vi "PositionControlTest.vi"() -> ()   [LabVIEW 2019]
uses:
  <vilib>/myRIO/Common/Instrument Driver Framework/myRIO v1.0/Encoder/typedefs/Encoder Count Direction Enum.ctl
  <vilib>/myRIO/Common/Instrument Driver Framework/myRIO v1.0/Encoder/typedefs/Encoder Signal Mode.ctl
  <vilib>/myRIO/Common/Instrument Driver Framework/myRIO v1.0/Encoder/typedefs/Encoder Channels Enum.ctl
  <vilib>/myRIO/Common/Instrument Driver Framework/Utilities/typedefs/Generic FPGA Reference.ctl
  <vilib>/myRIO/Common/Instrument Driver Framework/Utilities/typedefs/myRIO v1.0 Reference.ctl
  <vilib>/myRIO/Common/Instrument Driver Framework/Utilities/typedefs/Hardware Version Enum.ctl
  <vilib>/myRIO/Common/Instrument Driver Framework/Utilities/typedefs/myRIO Generic Hardware Reference.ctl
  <vilib>/myRIO/Instrument Drivers/Onboard IO/Encoder/typedefs/Encoder Reference.ctl
  <vilib>/myRIO/Instrument Drivers/Onboard IO/Encoder/Encoder.lvlib
  <vilib>/myRIO/Instrument Drivers/Onboard IO/Encoder/vis/Read.vi
  <vilib>/myRIO/Common/Instrument Driver Framework/myRIO v1.0/Encoder/typedefs/Encoder Configuration v1.0.ctl
  <vilib>/userdefined/High Color/nirio_resource_hc.ctl
  <vilib>/myRIO/Common/Instrument Driver Framework/myRIO v1.0/Encoder/vis/myRIO v1.1 Open Encoder.vi
  <vilib>/myRIO/Common/Instrument Driver Framework/myRIO v1.0/Encoder/vis/myRIO v1.0 Configure Encoder.vi
  <vilib>/myRIO/Instrument Drivers/Onboard IO/Encoder/vis/myRIO Encoder Open.xnode
  <vilib>/myRIO/Common/Instrument Driver Framework/Utilities/vis/Is FPGA Ref Available.vi
  <vilib>/myRIO/Express VI/Onboard IO/Encoder/Encoder Express VI.xnode
  <vilib>/Utility/file.llb/Write Delimited Spreadsheet (DBL).vi
  <vilib>/myRIO/Instrument Drivers/Utilities/Utilities.lvlib
panel:
  out "ref pos":dbl
  out "error out 2":errorcluster
  in  "Stop 2":bool
  out "Counter Direction":enum16{"Counting Up", "Counting Down"}(ring)
  out "Overflow?":bool
  in  "Reset Counter":bool
  out "actual pos":dbl
  out "Graph 2":cluster{dbl, dbl}(graph)
  in  "Frequency [Hz]":dbl=1000.0
  out "Duty Cycle":dbl=0.5
  in  "pos ref":dbl(slide) scale=-3.0..3.0
  in  "K":dbl format="%#_13g"
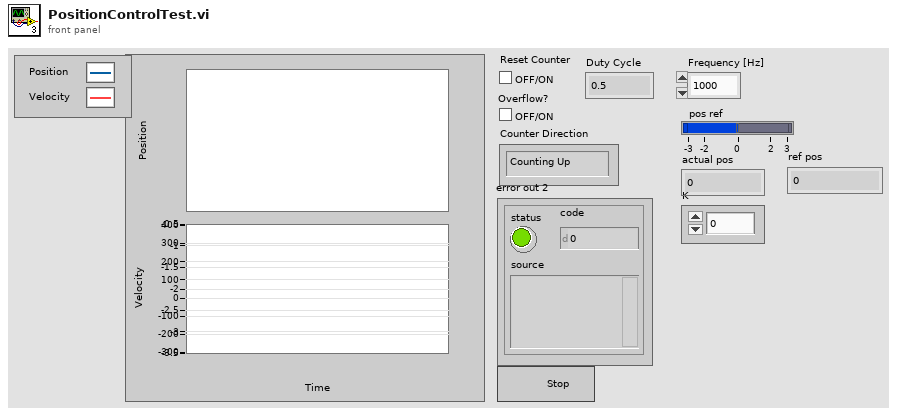
[diagram p1: front panel]
types:
  T1 = typedef "Encoder.lvlib/Encoder Reference.ctl" = cluster{"myRIO Reference":T2, "Encoder Channels Enum":T6}
  T2 = typedef "myRIO Generic Hardware Reference.ctl" = cluster{"myRIO Model":T3, "myRIO Hardware Reference":T4}
  T3 = typedef "Hardware Version Enum.ctl" = enum16{"Unknown", "myRIO-1900", "myRIO-1950", "roboRIO", "NI ELVIS RIO CM", "ELVIS III"}
  T4 = typedef "myRIO v1.0 Reference.ctl" = cluster{"Generic FPGA Reference":T5, "Allow multiple opens":bool}
  T5 = typedef "Generic FPGA Reference.ctl" = refnum<k20>
  T6 = typedef "Encoder Channels Enum.ctl" = enum16{"Not Connected", "C/ENC0", "C/ENC1", "A/ENC", "A/ENC0", "A/ENC1", "A/ENC2", "A/ENC3", "A/ENC4", "A/ENC5", "A/ENC6", "A/ENC7", "A/ENC8", "A/ENC9", "B/ENC", "B/ENC0", "B/ENC1", "B/ENC2", "B/ENC3", "B/ENC4", "B/ENC5", "B/ENC6", "B/ENC7", "B/ENC8", "B/ENC9", "DIO/ENC0", "DIO/ENC1", "DIO/ENC2", "DIO/ENC3", "DIO/ENC4"}
  T7 = typedef "Encoder Signal Mode.ctl" = enum16{"Quadrature phase signal", "Step and direction signal"}
  T8 = typedef "nirio_resource_hc.ctl" = tag
  T9 = typedef "Encoder Count Direction Enum.ctl" = enum16{"Counting Up", "Counting Down"}
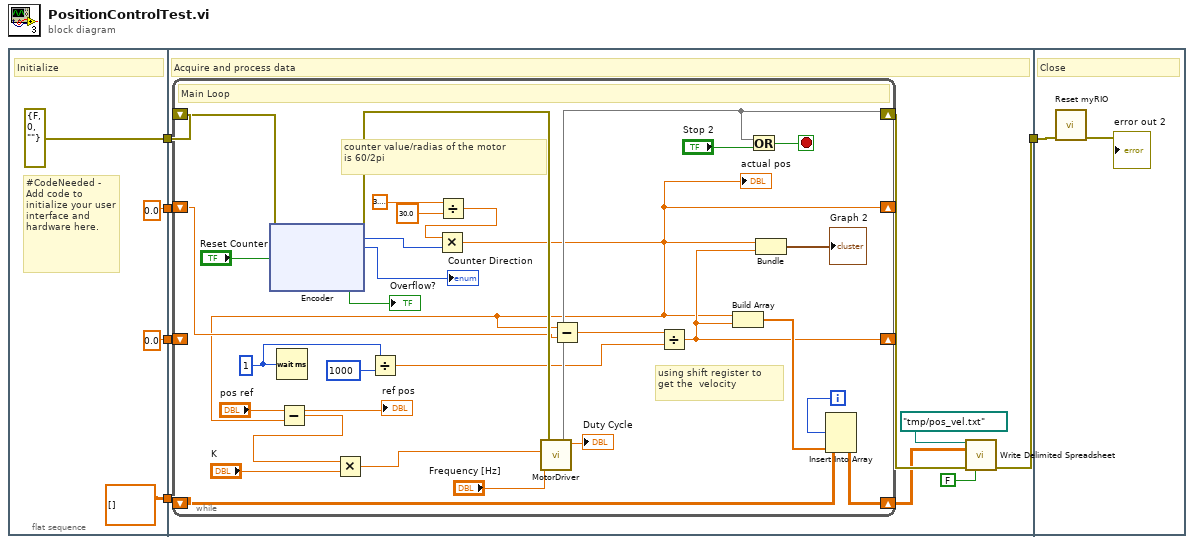
[diagram p0: block diagram]
diagram:
  n1 = flat-sequence {
    tunnel: [errorcluster {"status"=FALSE, "code"=0, "source"=""} ("error in (no error)")] -> w5
    tunnel: [0.0] -> w4
    tunnel: [dbl[][] [] ("array")] -> w3
    tunnel: [0.0] -> w2
    tunnel: w5 -> [w18]
    tunnel: [w13] -> w1
    tunnel: w4 -> [w17]
    tunnel: w3 -> [w16]
    tunnel: w2 -> [w10]
    tunnel: w1 -> [w96]
    frame #0 {
      # "#CodeNeeded - Add code to initialize your user interface and hardware here."
      # "Initialize"
    }
    frame #1 {
      # "Acquire and process data"
      n2 = while {
        shift-right: [w29] -> w14
        shift-left: w18 -> [w26]
        shift-right: [w22] -> _
        shift-left: w17 -> [w24]
        shift-right: [w34] -> w11
        shift-left: w16 -> [w19]
        shift-right: [w28] -> _
        shift-left: w10 -> [_]
        i -> [w35]
        stop <- w47 stop-if-true
        w41 = u32 1 ("milliseconds to wait")
        # "using shift register to\nget the  velocity"
        # "counter value/radias of the motor \nis 60/2pi"
        # "Main Loop"
        n3 = xnode "Encoder"("error in (no error)"=w26, "Reset Counter"="Reset Counter") -> ("error out"=w30:errorcluster, "Counter Value"=w38:i32, "Counter Direction"=→"Counter Direction":T9, "Overflow?"=→"Overflow?":bool)
        n4 = Wait (ms)(milliseconds to wait=w41) -> ()  [unwired: 1 out]
        n5 = Divide(x=w41, y=u32 1000) -> (x/y=w27:dbl)
        n6 = Divide(x=3.141592653589793, y=30.0) -> (x/y=w37:dbl)
        n7 = Multiply(x=w37, y=w38) -> (x*y=w22:dbl)
        "actual pos" <- w22
        n8 = Subtract(x="pos ref", y=w22) -> (x-y=w21:dbl)
        n9 = Multiply(x=w21, y="K") -> (x*y=w20:dbl)
        n10 = call "MotorDriver.vi"("error in (no error)"=w30, "Duty Cycle in"=w20, "Frequency [Hz]"="Frequency [Hz]") -> (0:w29, "Duty Cycle out"=→"Duty Cycle":dbl)  [unwired: 7 in]
        n11 = Subtract(x=w22, y=w24) -> (x-y=w39:dbl)
        n12 = Divide(x=w39, y=w27) -> (x/y=w28:dbl)
        n13 = Build Array(w22, w28) -> (w33:dbl[])
        n14 = Or(x=w29, y="Stop 2") -> (x .or. y?=w47:bool)
        n15 = Bundle(w22, w28) -> (→"Graph 2":cluster{dbl, dbl})  [unwired: 1 in]
        n16 = Insert Into Array(array=w19, index (row)=w35, new element=w33) -> (w34:dbl[][])  [unwired: 1 in]
        "ref pos" <- "pos ref"
      }
      n17 = call-poly <vilib>:"Write Delimited Spreadsheet.vi"("file path (dialog if empty)"=path "/tmp/pos_vel.txt", "2D data"=w11, "error in (no error)"=w14, "transpose? (no:F)"=FALSE) -> ("error out"=w13:errorcluster)  [unwired: 10 in, 1 out]
    }
    frame #2 {
      # "Close"
      n18 = call <vilib>:"Reset myRIO.vi"("error in (no error)"=w96) -> ("error out"=→"error out 2":errorcluster)  [unwired: 10 in]
    }
  }
